vi "Create LVClass Copy.vi"(5 "Override existing":bool, 6 "New Name":string, 7 "Use Relative":bool, 8 "error in (no error)":errorcluster, 9 "New Path":string, 10 "Source Class Path":path, 11 "Application in":refnum<vi>) -> (0 "error out":errorcluster, 2 "Copy Class Path out":path, 3 "Application reference out":refnum<vi>)   [LabVIEW 2019, in "gRPC Template Creation Utility.lvlib"]
uses:
  gRPC Template Creation Utility.lvlib
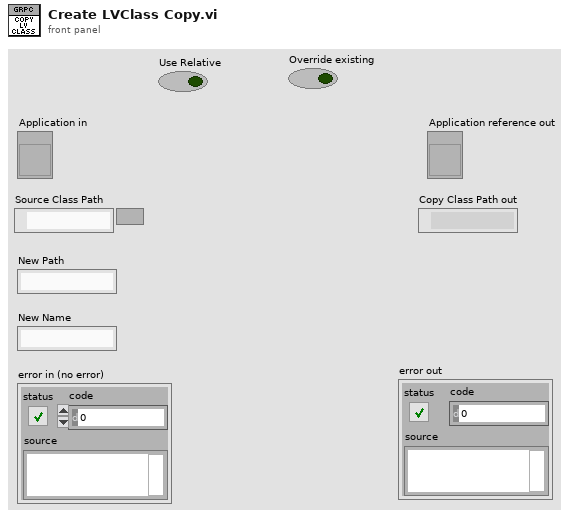
[diagram p1: front panel]
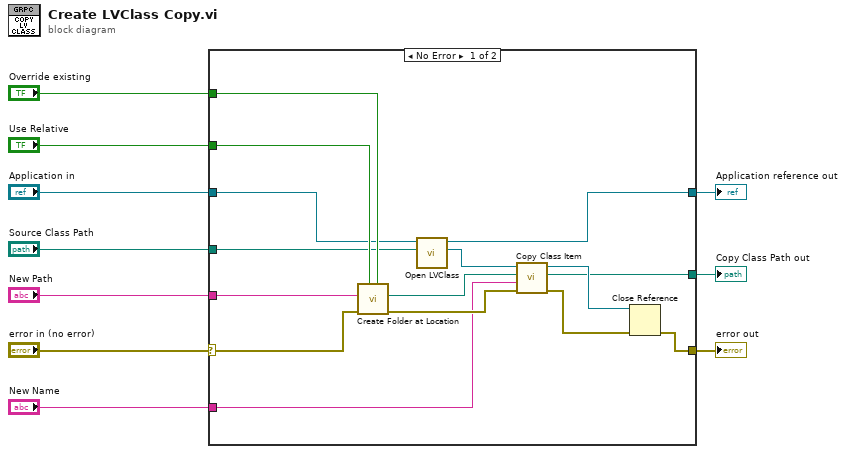
[diagram p0: block diagram]
diagram:
  n1 = case shown="No Error" "error in (no error)" {
    selector: "error in (no error)" -> [w11 w27]
    tunnel: "Use Relative" -> [w25 _]
    tunnel: "Override existing" -> [w24 _]
    tunnel: "Application in" -> [w23 w26]
    tunnel: "Source Class Path" -> [w22 _]
    tunnel: "New Name" -> [w20 _]
    tunnel: "New Path" -> [w18 _]
    tunnel: [w16 w26] -> w4
    tunnel: [w13 _] -> w3
    tunnel: [w12 w27] -> w2
    frame No Error {
      n2 = call "Create Folder at Location.vi"("Override existing (F)"=w24, "Use Relative (F)"=w25, "Error In"=w11, "Path"=w18) -> ("Error Out"=w21:errorcluster, "Full path out"=w19:path)  [unwired: 5 in, 1 out]
      n3 = call "Open LVClass.vi"("Full Path"=w22, "Application reference in"=w23) -> ("LVClass out"=w17:refnum<vi>, "Application reference out"=w16:refnum<vi>)  [unwired: 7 in, 1 out]
      n4 = call "Copy Class Item.vi"("error in (no error)"=w21, "New Name"=w20, "Full path in"=w19, "LVClassLibrary in"=w17) -> ("error out"=w15:errorcluster, "New Class Path out"=w13:path, "LVClassLibrary out"=w14:refnum<vi>)  [unwired: 5 in]
      n5 = Close Reference(reference=w14, error in (no error)=w15) -> (error out=w12:errorcluster)
    }
    frame Error {
    }
  }
  "Copy Class Path out" <- w3
  "Application reference out" <- w4
  "error out" <- w2
